vi "Close.vi"(8 "error in (no error)":errorcluster, 11 "Hioki 9002 in":refnum<class "Hioki 9002.lvclass">) -> (0 "error out":errorcluster, 3 "Hioki 9002 out":refnum<class "Hioki 9002.lvclass">)   [LabVIEW 2025, in "Switch.lvlib" / "Hioki 9002.lvclass"]
uses:
  Hioki 9002.lvclass
  Hioki 9002.lvclass/Hioki 9002.ctl
  <instrlib>/HIOKI SW100X Series/HIOKI SW100X Series.lvlib
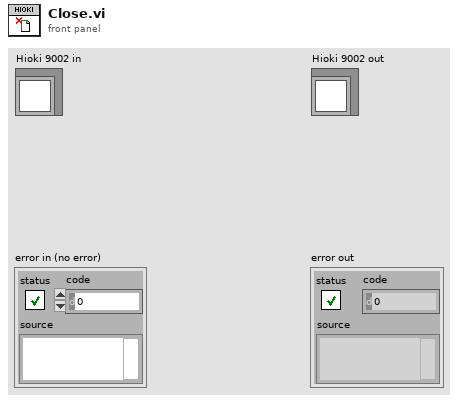
[diagram p1: front panel]
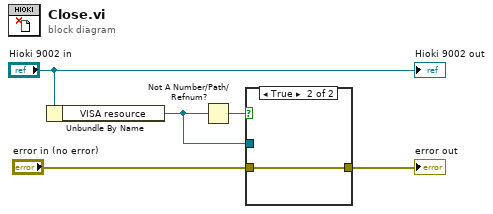
[diagram p0: block diagram]
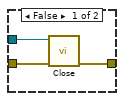
[diagram p2: hidden frame]
diagram:
  n1 = Unbundle By Name("Hioki 9002 in") -> ("VISA resource"=w5:refnum<visa-resource-name>)
  n2 = Not A Number/Path/Refnum?(number/path/refnum=w5) -> (NaN/Path/Refnum?=w4:bool)
  n3 = case shown="True" w4 {
    tunnel: "error in (no error)" -> [w7 w9]
    tunnel: [w6 w9] -> w1
    tunnel: w5 -> [w8 _]
    frame False {
      n4 = call <instrlib>:"Close.vi"("error in (no error)"=w7, "VISA resource name"=w8) -> ("error out"=w6:errorcluster)  [unwired: 9 in]
    }
    frame True {
    }
  }
  "error out" <- w1
  "Hioki 9002 out" <- "Hioki 9002 in"
